vi "Navigation_Sensors_G.vi"(8 "Speed":dbl, 9 "car_theta":dbl, 10 "car_pos":dbl[](array[numeric]), 11 "Look_Ahead":dbl) -> (1 "Theta_1":dbl, 2 "d":dbl, 3 "Theta_2":dbl)   [LabVIEW 2018]
uses:
  <vilib>/Simulation/Scripting/Companion Diagram/SimConfigNode/SimParams.ctl
  <vilib>/Simulation/Scripting/Companion Diagram/SimConfigNode/_simSolvers.ctl
  <vilib>/Simulation/Implementation/Shared/SIMSCR Execution Mode.ctl
  <vilib>/Simulation/Param Hierarchy/Typedefs/SIMPH Param Control Actions.ctl
  <vilib>/Simulation/Implementation/Shared/NILVSim_FinalizeModel.vi
  <vilib>/Utility/error.llb/Clear Errors.vi
  <vilib>/Simulation/SignalArithmetic/Implementation/NILVSim Gain.llb/SIM Gain (scalar).vi
  <vilib>/Simulation/Utility/Implementation/NILVSim Memory.llb/NILVSim Memory (core).vi
  <vilib>/Simulation/Implementation/Shared/NILVSim_Manager.vi
  <vilib>/Simulation/Implementation/Shared/NILVSIM_BeginStep.vi
  <vilib>/Simulation/Implementation/Shared/NILVSim_ParamChanged.vi
  <vilib>/Simulation/Implementation/Shared/SIM Unbundle Sim Info.vi
  <vilib>/Simulation/Implementation/Shared/SIMSH Read Queue.vi
  <vilib>/Simulation/Implementation/Shared/NILVSim_Initialize.vi
  <vilib>/Simulation/Utility/Implementation/NILVSim Get Time and IsAcceptedStep.vi
  <vilib>/Simulation/Implementation/Shared/NILVSim_GetModelError.vi
  <vilib>/Simulation/Implementation/Shared/SIM SimErrorHandler.vi
  <vilib>/Simulation/Implementation/Shared/SIM Bundle Sim Info.vi
  <vilib>/Simulation/Scripting/Companion Diagram/SimConfigNode/SimDog.xnode
  <vilib>/Simulation/Implementation/XNodeFramework/SimXNode/SimX.xnode
  <vilib>/Simulation/Implementation/Shared/NI_SIM_Implementation.lvlib
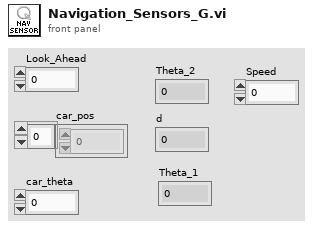
[diagram p1: front panel]
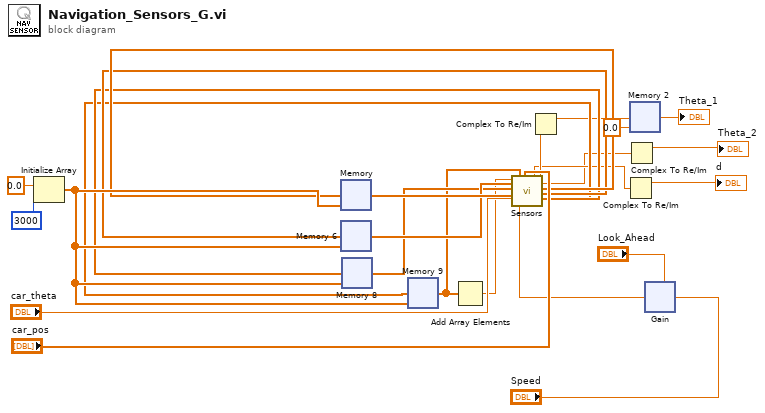
[diagram p0: block diagram]
diagram:
  n1 = Initialize Array(0.0 ("element"), 3000 ("dimension size")) -> (w25:dbl[])
  n2 = xnode ("Gain")("gain"="Look_Ahead", "input"="Speed") -> ("output"=w11:dbl)  [unwired: 2 in]
  n3 = xnode ("Memory")("input"=w15, "initial value"=w25) -> ("output"=w22:dbl[])  [unwired: 4 in]
  n4 = xnode ("Memory 6")("input"=w14, "initial value"=w25) -> ("output"=w21:dbl[])  [unwired: 4 in]
  n5 = xnode ("Memory 8")("input"=w13, "initial value"=w25) -> ("output"=w20:dbl[])  [unwired: 4 in]
  n6 = xnode ("Memory 9")("input"=w12, "initial value"=w25) -> ("output"=w17:dbl[])  [unwired: 4 in]
  n7 = Add Array Elements(numeric array=w17) -> (sum=w18:dbl)
  n8 = call "Sensors.vi"("total_length"=w18, "x"=w21, "y"=w20, "theta"=w22, "car_theta"="car_theta", "segment_distance"=w17, "Look_ahead_distance"=w11, "car_pos"="car_pos") -> ("min_dist"=w6:cdb, "segment_distance"=w12:cdb[], "Theta_1"=w8:cdb, "Theta_2"=w4:cdb, "theta"=w15:dbl[], "x"=w14:dbl[], "y"=w13:dbl[])  [unwired: 4 in, 1 out]
  n9 = Complex To Re/Im(x + iy=w8) -> (x=w7:dbl)  [unwired: 1 out]
  n10 = Complex To Re/Im ("Complex To Re/Im 2")(x + iy=w6) -> (x=→"d":dbl)  [unwired: 1 out]
  n11 = Complex To Re/Im ("Complex To Re/Im 3")(x + iy=w4) -> (x=→"Theta_2":dbl)  [unwired: 1 out]
  n12 = xnode ("Memory 2")("input"=w7, "initial value"=0.0) -> ("output"=→"Theta_1":dbl)  [unwired: 4 in]
